vi "changeStatus.vi"(8 "error in (no error)":errorcluster, 10 "status":T1(ring), 11 "HWController in":refnum<class "HWController.lvclass">) -> (0 "error out":errorcluster, 3 "HWController out":refnum<class "HWController.lvclass">)   [LabVIEW 2011, in "Hardware.lvlib" / "HWControllers.lvlib" / "HWController.lvclass"]
uses:
  HWController.lvclass
  HWController.lvclass/HWController.ctl
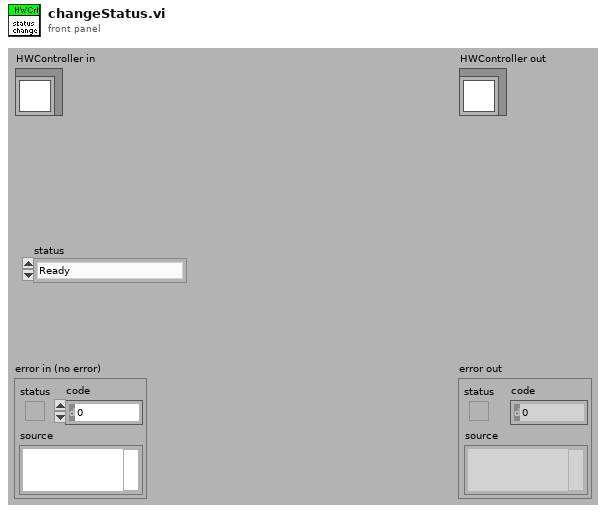
[diagram p1: front panel]
types:
  T1 = enum16{"Ready", "Compiling", "Configured", "Running", "Stopping", "Unresolved Error"}
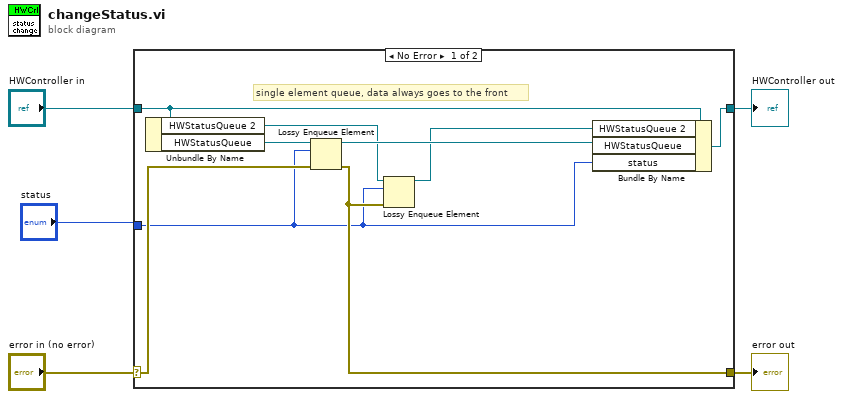
[diagram p0: block diagram]
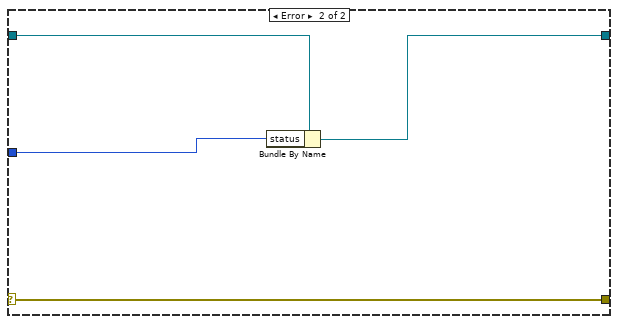
[diagram p2: hidden frame]
diagram:
  n1 = case shown="No Error" "error in (no error)" {
    selector: "error in (no error)" -> [w11 w18]
    tunnel: [w9 w18] -> w4
    tunnel: [w14 w16] -> w2
    tunnel: "HWController in" -> [w13 w17]
    tunnel: "status" -> [w6 w15]
    frame No Error {
      # "single element queue, data always goes to the front"
      n2 = Unbundle By Name(w13) -> ("HWStatusQueue 2"=w8:refnum<queue>, "HWStatusQueue"=w12:refnum<queue>)
      n3 = Lossy Enqueue Element(queue=w12, element=w6, error in (no error)=w11) -> (queue out=w10:refnum<queue>, error out=w9:errorcluster)  [unwired: 2 out]
      n4 = Lossy Enqueue Element(queue=w8, element=w6, error in (no error)=w9) -> (queue out=w7:refnum<queue>)  [unwired: 3 out]
      n5 = Bundle By Name(cluster=w13, "HWStatusQueue 2"=w7, "HWStatusQueue"=w10, "status"=w6) -> (w14:refnum<class "HWController.lvclass">)
    }
    frame Error {
      n6 = Bundle By Name(cluster=w17, "status"=w15) -> (w16:refnum<class "HWController.lvclass">)
    }
  }
  "error out" <- w4
  "HWController out" <- w2
